vi "Unlock all VIs.vi"(1 "Path":path) -> ()   [LabVIEW 2020, in "LeMaal.lvlib"]
uses:
  LeMaal.lvlib
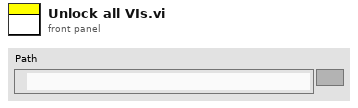
[diagram p1: front panel]
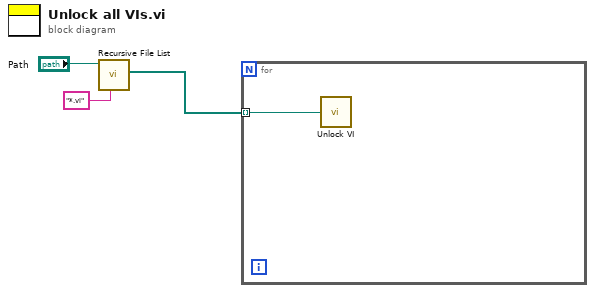
[diagram p0: block diagram]
diagram:
  n1 = call <vilib>:"Recursive File List.vi"("pattern"="*.vi", "Folder Path"="Path") -> ("All Files in Dir"=w1:path[])  [unwired: 5 in, 4 out]
  n2 = for {
    tunnel: w1 -> [w4] mode=indexing
    n3 = call "Unlock VI.vi"("VI File"=w4) -> ()  [unwired: 1 out]
  }
